vi "Get Frame Rate.vi"(8 "error in (no error)":errorcluster, 11 "Camera in":refnum<class "Camera.lvclass">) -> (0 "error out":errorcluster, 2 "Pixel Format":string, 3 "Camera":refnum<class "Camera.lvclass">)   [LabVIEW 2020, in "Camera.lvclass"]
uses:
  Camera.lvclass
  Camera.lvclass/Camera.ctl
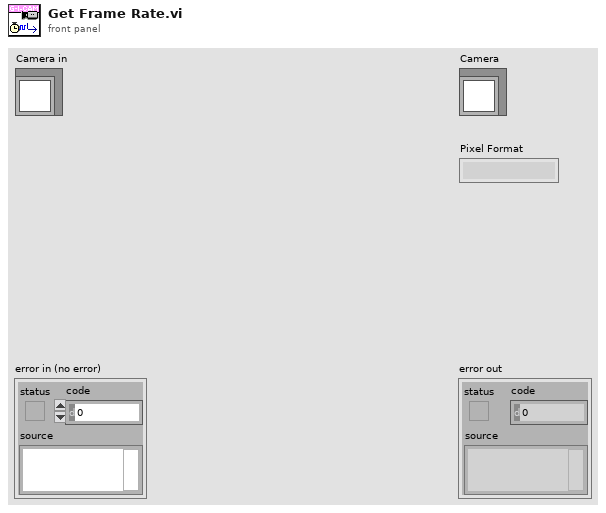
[diagram p1: front panel]
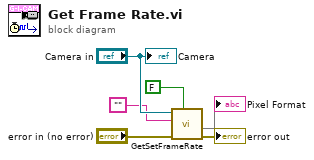
[diagram p0: block diagram]
diagram:
  n1 = call "GetSetFrameRate.vi"("Set?"=FALSE, "error in (no error)"="error in (no error)", "Value in"="", "Camera in"="Camera in") -> ("error out"=→"error out":errorcluster, 1:→"Pixel Format")  [unwired: 5 in, 1 out]
  "Camera" <- "Camera in"
